vi "PWM_INIT.vi"(2 "error in (no error)":errorcluster, 3 "Period":i32 min=0 max=65535, 4 "Duty":i32 min=0 max=1023, 5 "VISA resource name":refnum<visa-resource-name>) -> (0 "error out":errorcluster, 1 "VISA resource Quit":refnum<visa-resource-name>)   [LabVIEW 2011]
panel:
  out "unsigned byte array":u8[](array[numeric])
  out "return count":u32
  out "Read PWM_INIT command":u8[](array[numeric])
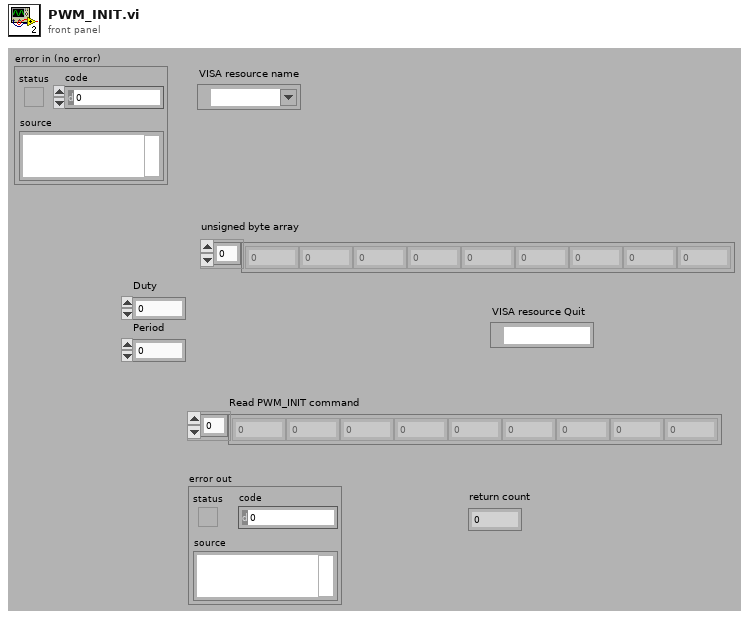
[diagram p1: front panel]
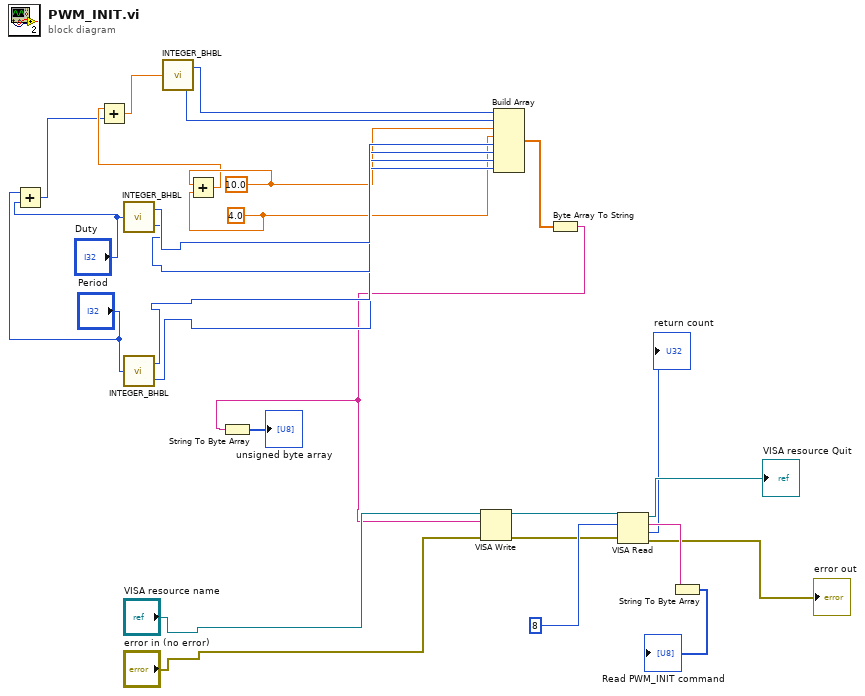
[diagram p0: block diagram]
diagram:
  w9 = 4.0 ("element")
  w8 = 10.0 ("element")
  n1 = Add(x="Period", y="Duty") -> (x+y=w6:i32)
  n2 = call "INTEGER_BHBL.vi"("int16"="Duty") -> ("Lvalue"=w16:u8, "HValue"=w17:u8)
  n3 = call "INTEGER_BHBL.vi"("int16"="Period") -> ("Lvalue"=w14:u8, "HValue"=w15:u8)
  n4 = Add(x=w8, y=w9) -> (x+y=w7:dbl)
  n5 = Add(x=w7, y=w6) -> (x+y=w5:dbl)
  n6 = call "INTEGER_BHBL.vi"("int16"=w5) -> ("Lvalue"=w3:u8, "HValue"=w4:u8)
  n7 = Build Array(w4, w3, w8, w9, w17, w16, w15, w14) -> (w19:dbl[])
  n8 = Byte Array To String(unsigned byte array=w19) -> (string=w2:string)
  n9 = String To Byte Array(string=w2) -> (unsigned byte array=→"unsigned byte array":u8[])
  n10 = VISA Write(VISA resource name="VISA resource name", write buffer=w2, error in (no error)="error in (no error)") -> (VISA resource name out=w20:refnum<visa-resource-name>, error out=w22:errorcluster)  [unwired: 1 out]
  n11 = VISA Read(VISA resource name=w20, byte count=u32 8, error in (no error)=w22) -> (VISA resource name out=→"VISA resource Quit":refnum<visa-resource-name>, read buffer=w25:string, return count=→"return count":u32, error out=→"error out":errorcluster)
  n12 = String To Byte Array(string=w25) -> (unsigned byte array=→"Read PWM_INIT command":u8[])
